vi "Assert ExcuseNotes MultiTable.vi"() -> ()   [LabVIEW 2015, in "ExcuseNotesHandler.lvclass"]
uses:
  ExcuseNotesHandler.lvclass
  <vilib>/Utility/miscctls.llb/LVPoint32TypeDef.ctl
  <vilib>/Utility/miscctls.llb/LVPositionTypeDef.ctl
panel:
  out "Coords":T1
  in  "是否同意":bool
  in  "Stop":bool
  in  "Table Control":string[][](table)
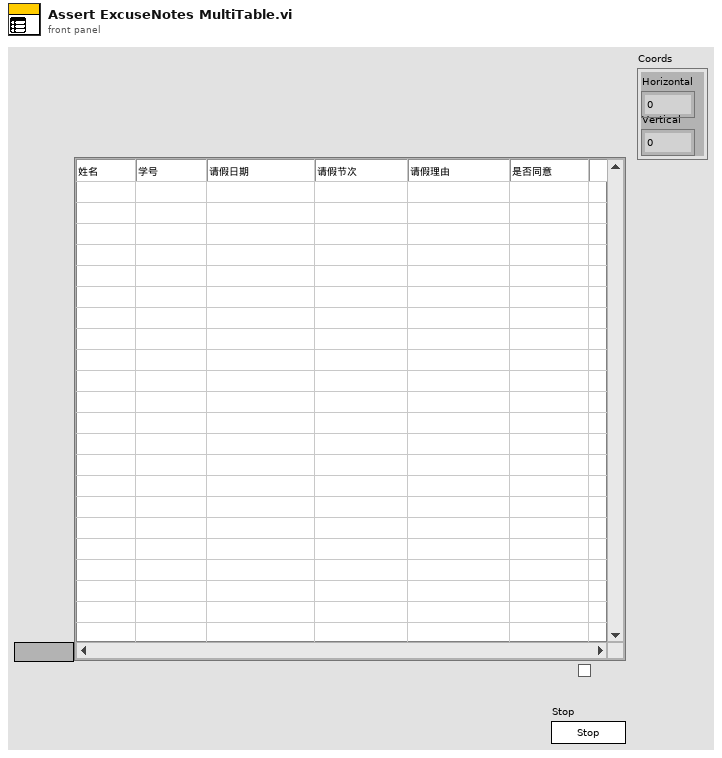
[diagram p1: front panel]
types:
  T1 = typedef "LVPoint32TypeDef.ctl" = cluster{"Horizontal":i32, "Vertical":i32}
  T2 = typedef "LVPositionTypeDef.ctl" = cluster{"Left":i32, "Top":i32}
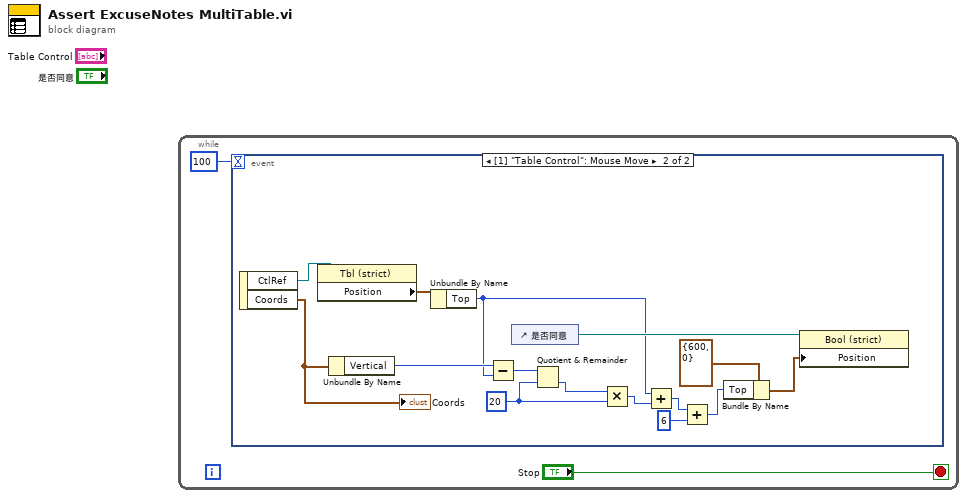
[diagram p0: block diagram]
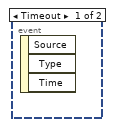
[diagram p2: hidden frame]
diagram:
  n1 = while {
    stop <- "Stop" stop-if-true
    n2 = event shown="[1] \"Table Control\": Mouse Move" {
      selector: _ -> [_ _]
      dyn-events: _ -> [_ _]
      timeout: 100 -> [_ _]
      event Timeout {
        n3 = event-data() -> ()  [unwired: 1 in, 3 out]
      }
      event "Table Control": Mouse Move {
        w12 = 20 ("y")
        n4 = event-data() -> ("CtlRef"=w17:refnum<vi>, "Coords"=w16:T1)  [unwired: 1 in]
        "Coords" <- w16
        n5 = property class="Tbl (strict)"(reference=w17) -> ("Position"=w15:T2)  [unwired: 1 in, 2 out]
        n6 = Unbundle By Name(w16) -> ("Vertical"=w14:i32)
        n7 = Unbundle By Name(w15) -> ("Top"=w7:i32)
        n8 = Subtract(x=w14, y=w7) -> (x-y=w13:i32)
        n9 = control-ref of="是否同意"() -> (w11:refnum<vi>)
        n10 = Quotient & Remainder(x=w13, y=w12) -> (floor(x/y)=w6:i32)  [unwired: 1 out]
        n11 = Multiply(x=w6, y=w12) -> (x*y=w8:i32)
        n12 = Add(x=w7, y=w8) -> (x+y=w5:i32)
        n13 = Add(x=w5, y=6) -> (x+y=w4:i32)
        n14 = Bundle By Name(cluster=T2 {"Left"=600, "Top"=0} ("Position"), "Top"=w4) -> (w9:T2)
        n15 = property class="Bool (strict)"(reference=w11, "Position"=w9) -> ()  [unwired: 1 in, 2 out]
      }
    }
  }
